vi "Lab5.vi"() -> ()   [LabVIEW 2014]
panel:
  in  "Corn":bool
  in  "Fox":bool
  in  "Hen":bool
  out "Alarm":bool
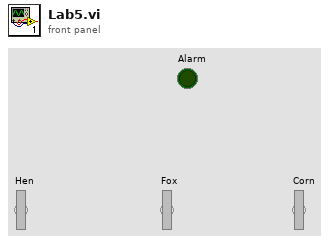
[diagram p1: front panel]
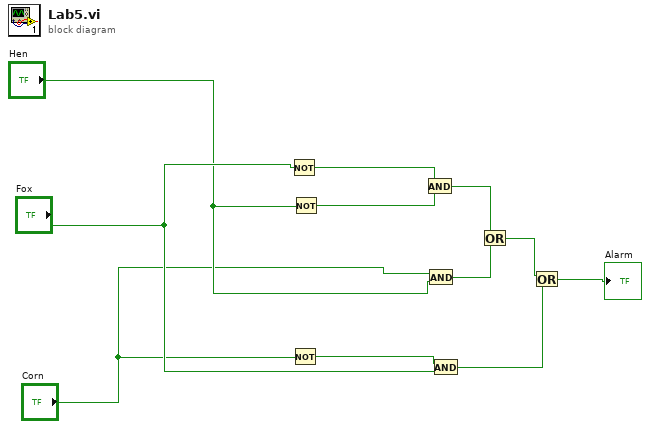
[diagram p0: block diagram]
diagram:
  n1 = Not(x="Fox") -> (.not. x?=w10:bool)
  n2 = Not(x="Corn") -> (.not. x?=w4:bool)
  n3 = Not(x="Hen") -> (.not. x?=w11:bool)
  n4 = And(x=w10, y=w11) -> (x .and. y?=w9:bool)
  n5 = And(x="Corn", y="Hen") -> (x .and. y?=w8:bool)
  n6 = And(x=w4, y="Fox") -> (x .and. y?=w5:bool)
  n7 = Or(x=w9, y=w8) -> (x .or. y?=w6:bool)
  n8 = Or(x=w6, y=w5) -> (x .or. y?=→"Alarm":bool)
